vi "Scaling Coefficients from INI.vi"(8 "error in":errorcluster, 11 "Config Refnum in":T1) -> (0 "error out":errorcluster, 3 "Config Refnum out":T1, 4 "Scaling Coefficients":T2)   [LabVIEW 2018]
uses:
  Controls/Scaling Coefficients Cluster.ctl
  Controls/Scaling Coefficients Measurements.ctl
  Controls/Scaling Coefficients Setpoints.ctl
  <vilib>/Utility/config.llb/Config Data RefNum.ctl
  <vilib>/Utility/config.llb/Read Key (Double).vi
  <vilib>/Utility/config.llb/NI_LVConfig.lvlib
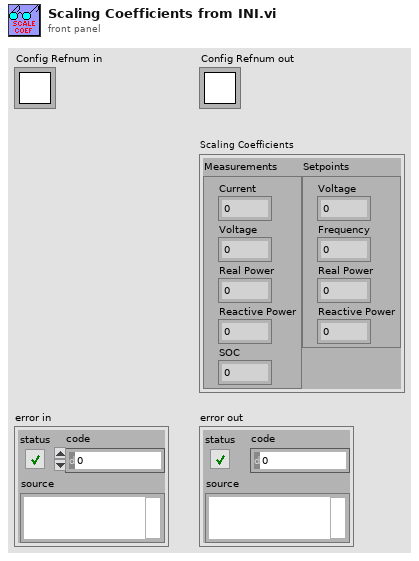
[diagram p1: front panel]
types:
  T1 = typedef "NI_LVConfig.lvlib/Config Data RefNum.ctl" = refnum<k1>
  T2 = typedef "Scaling Coefficients Cluster.ctl" = cluster{"Measurements":T3, "Setpoints":T4}
  T3 = typedef "Scaling Coefficients Measurements.ctl" = cluster{"Current":dbl, "Voltage":dbl, "Real Power":dbl, "Reactive Power":dbl, "SOC":dbl}
  T4 = typedef "Scaling Coefficients Setpoints.ctl" = cluster{"Voltage":dbl, "Frequency":dbl, "Real Power":dbl, "Reactive Power":dbl}
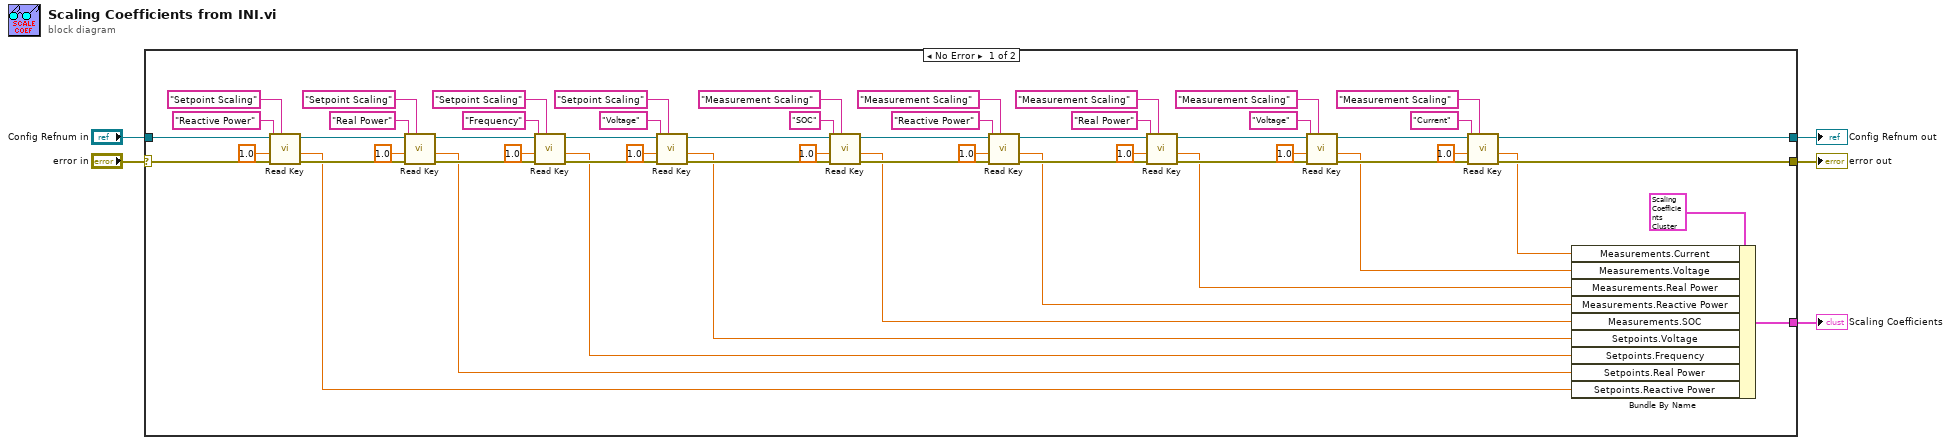
[diagram p0: block diagram]
diagram:
  n1 = case shown="No Error" "error in" {
    selector: "error in" -> [w58 w65]
    tunnel: [w63 _] -> w5
    tunnel: [w62 w65] -> w4
    tunnel: [w61 w64] -> w3
    tunnel: "Config Refnum in" -> [w57 w64]
    frame No Error {
      n2 = call-poly <vilib>:"Read Key.vi"("section"="Setpoint Scaling", "error in (no error)"=w58, "default value"=1.0, "key"="Reactive Power", "refnum"=w57) -> ("error out"=w60:errorcluster, "value"=w14:dbl, "refnum out"=w59:T1)  [unwired: 3 in, 1 out]
      n3 = call-poly <vilib>:"Read Key.vi"("section"="Setpoint Scaling", "error in (no error)"=w60, "default value"=1.0, "key"="Real Power", "refnum"=w59) -> ("error out"=w49:errorcluster, "value"=w13:dbl, "refnum out"=w48:T1)  [unwired: 3 in, 1 out]
      n4 = call-poly <vilib>:"Read Key.vi"("section"="Setpoint Scaling", "error in (no error)"=w49, "default value"=1.0, "key"="Frequency", "refnum"=w48) -> ("error out"=w51:errorcluster, "value"=w12:dbl, "refnum out"=w50:T1)  [unwired: 3 in, 1 out]
      n5 = call-poly <vilib>:"Read Key.vi"("section"="Setpoint Scaling", "error in (no error)"=w51, "default value"=1.0, "key"="Voltage", "refnum"=w50) -> ("error out"=w53:errorcluster, "value"=w11:dbl, "refnum out"=w52:T1)  [unwired: 3 in, 1 out]
      n6 = call-poly <vilib>:"Read Key.vi"("section"="Measurement Scaling", "error in (no error)"=w53, "default value"=1.0, "key"="SOC", "refnum"=w52) -> ("error out"=w40:errorcluster, "value"=w10:dbl, "refnum out"=w36:T1)  [unwired: 3 in, 1 out]
      n7 = call-poly <vilib>:"Read Key.vi"("section"="Measurement Scaling", "error in (no error)"=w40, "default value"=1.0, "key"="Reactive Power", "refnum"=w36) -> ("error out"=w41:errorcluster, "value"=w9:dbl, "refnum out"=w37:T1)  [unwired: 3 in, 1 out]
      n8 = call-poly <vilib>:"Read Key.vi"("section"="Measurement Scaling", "error in (no error)"=w41, "default value"=1.0, "key"="Real Power", "refnum"=w37) -> ("error out"=w42:errorcluster, "value"=w8:dbl, "refnum out"=w38:T1)  [unwired: 3 in, 1 out]
      n9 = call-poly <vilib>:"Read Key.vi"("section"="Measurement Scaling", "error in (no error)"=w42, "default value"=1.0, "key"="Voltage", "refnum"=w38) -> ("error out"=w43:errorcluster, "value"=w7:dbl, "refnum out"=w39:T1)  [unwired: 3 in, 1 out]
      n10 = call-poly <vilib>:"Read Key.vi"("section"="Measurement Scaling", "error in (no error)"=w43, "default value"=1.0, "key"="Current", "refnum"=w39) -> ("error out"=w62:errorcluster, "value"=w6:dbl, "refnum out"=w61:T1)  [unwired: 3 in, 1 out]
      n11 = Bundle By Name(cluster=T2 {"Measurements"={"Current"=0.0, "Voltage"=0.0, "Real Power"=0.0, "Reactive Power"=0.0, "SOC"=0.0}, "Setpoints"={"Voltage"=0.0, "Frequency"=0.0, "Real Power"=0.0, "Reactive Power"=0.0}} ("Scaling Coefficients"), "Measurements.Current"=w6, "Measurements.Voltage"=w7, "Measurements.Real Power"=w8, "Measurements.Reactive Power"=w9, "Measurements.SOC"=w10, "Setpoints.Voltage"=w11, "Setpoints.Frequency"=w12, "Setpoints.Real Power"=w13, "Setpoints.Reactive Power"=w14) -> (w63:T2)
    }
    frame Error {
    }
  }
  "Scaling Coefficients" <- w5
  "error out" <- w4
  "Config Refnum out" <- w3
